vi "Read Shared Resources.vi"(8 "error in (no error)":errorcluster, 11 "LangFile in":refnum<class "Resource Data.lvclass">) -> (0 "error out":errorcluster, 2 "Shared Resources []":T1[](array[typedef]), 3 "LangFile out":refnum<class "Resource Data.lvclass">)   [LabVIEW 2013, in "SET Project Data.lvlib" / "Resource Data.lvclass"]
uses:
  Resource Data.lvclass
  Types/ProjFile_Resource Entry.ctl
  Resource Data.lvclass/Resource Data.ctl
  SET Project Data.lvlib
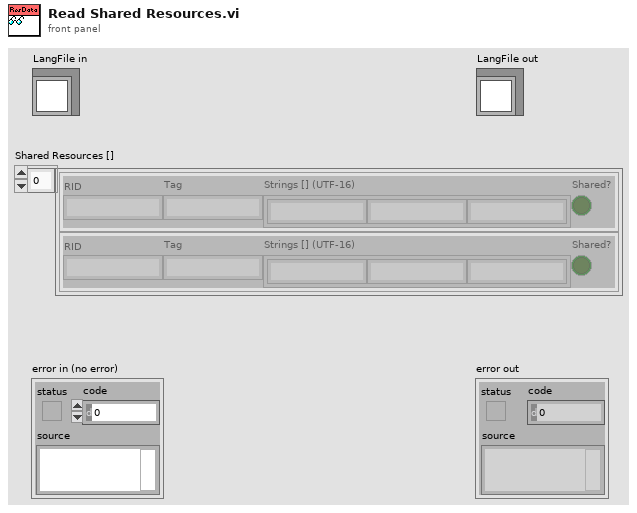
[diagram p1: front panel]
types:
  T1 = typedef "SET Project Data.lvlib/ProjFile_Resource Entry.ctl" = cluster{"RID":string, "Tag":string, "Strings [] (UTF-16)":string[], "Shared?":bool}
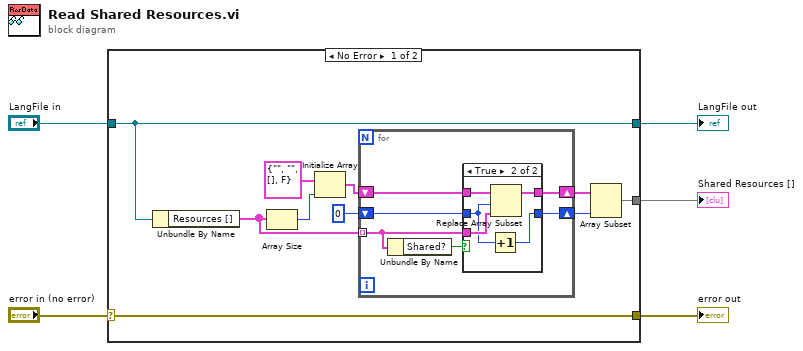
[diagram p0: block diagram]
diagram:
  n1 = case shown="No Error" "error in (no error)" {
    selector: "error in (no error)" -> [w15 w29]
    tunnel: [w15 w29] -> w4
    tunnel: [w14 w30] -> w2
    tunnel: "LangFile in" -> [w14 w30]
    tunnel: [w6 _] -> w1
    frame No Error {
      n2 = Unbundle By Name(w14) -> ("Resources []"=w11:T1[])
      n3 = Array Size(array=w11) -> (size(s)=w13:i32)
      n4 = Initialize Array(T1 {"RID"="", "Tag"="", "Strings [] (UTF-16)"=[], "Shared?"=FALSE} ("Resource"), w13) -> (w10:T1[])
      n5 = for {
        tunnel: w11 -> [w20] mode=indexing
        shift-right: [w17] -> w8
        shift-left: w10 -> [w19]
        shift-right: [w16] -> w7
        shift-left: 0 -> [w18]
        n6 = Unbundle By Name(w20) -> ("Shared?"=w21:bool)
        n7 = case shown="True" w21 {
          tunnel: w20 -> [_ w27]
          tunnel: w19 -> [w22 w28]
          tunnel: w18 -> [w23 w25]
          tunnel: [w22 w26] -> w17
          tunnel: [w23 w24] -> w16
          frame False {
          }
          frame True {
            n8 = Increment(x=w25) -> (x+1=w24:i32)
            n9 = Replace Array Subset(array=w28, new element=w27, index=w25) -> (w26:T1[])
          }
        }
      }
      n10 = Array Subset(array=w8, length=w7) -> (w6:T1[])  [unwired: 1 in]
    }
    frame Error {
    }
  }
  "error out" <- w4
  "LangFile out" <- w2
  "Shared Resources []" <- w1
